vi "setUp.vi"(8 "error in (no error)":errorcluster, 11 "TestConfigurationFileBinding In":refnum<class "TestPersistToDiskTransport.lvclass">) -> (0 "error out":errorcluster, 3 "TestConfigurationFileBinding Out":refnum<class "TestPersistToDiskTransport.lvclass">)   [LabVIEW 2017, in "TestPersistToDiskTransport.lvclass"]
doc: "setUp runs prior to the test method during test execution. Use this method to initialize any object data required by your tests."
uses:
  TestPersistToDiskTransport.lvclass
  C:/Program Files (x86)/National Instruments/LabVIEW 2017/vi.lib/addons/_JKI Toolkits/VI Tester/TestCase.llb/TestCase.lvclass
  <vilib>/Utility/sysdir.llb/System Directory Type.ctl
  TestPersistToDiskTransport.lvclass/TestPersistToDiskTransport.ctl
  <vilib>/addons/_JKI Toolkits/VI Tester/TestCase.llb/TestCase.lvclass
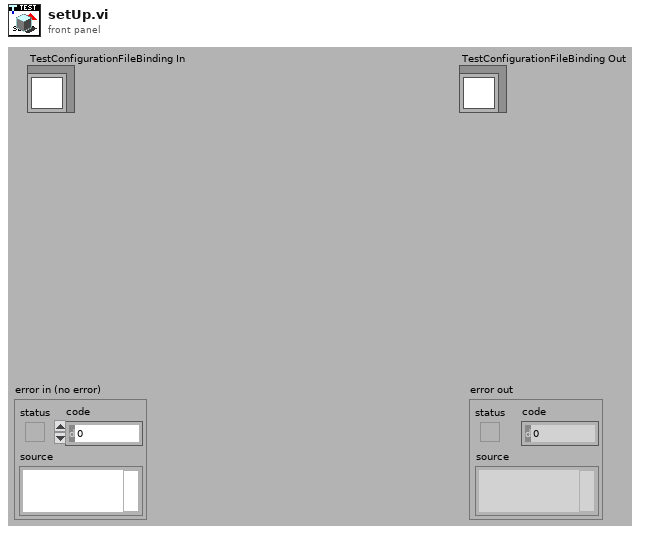
[diagram p1: front panel]
types:
  T1 = typedef "System Directory Type.ctl" = i32
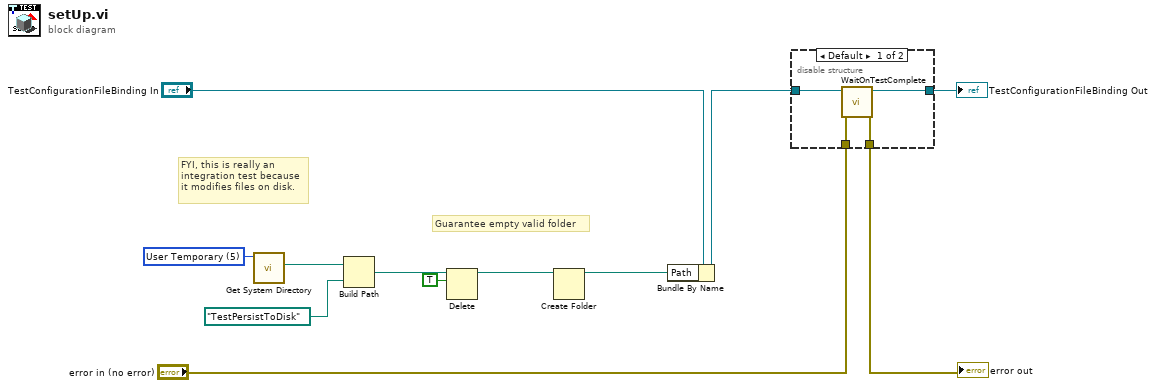
[diagram p0: block diagram]
diagram:
  w7 = T1 5 items=["User Home"=0, "User Desktop"=1, "User Documents"=2, "User Application Data"=3, "User Preferences"=4, "User Temporary"=5, "Public Documents"=6, "Public Application Data"=7, "Public Preferences"=8, "Public Cache"=13, "System Core Libraries"=9, "System Installed Libraries"=10, "Application Files"=11, "Boot Volume Root"=12] ("system directory type")
  # "Guarantee empty valid folder"
  # "FYI, this is really an\nintegration test because\nit modifies files on disk."
  n1 = call <vilib>:"Get System Directory.vi"("system directory type"=w7) -> ("system directory"=w6:path)  [unwired: 10 in]
  n2 = Build Path(base path=w6, name or relative path=path "TestPersistToDisk") -> (appended path=w4:path)
  n3 = Delete(path (use dialog)=w4, entire hierarchy (F)=TRUE) -> (deleted path=w2:path)  [unwired: 3 in, 2 out]
  n4 = Create Folder(path (use dialog)=w2) -> (created path=w3:path)  [unwired: 2 in, 2 out]
  n5 = Bundle By Name(cluster="TestConfigurationFileBinding In", "Path"=w3) -> (w8:refnum<class "TestPersistToDiskTransport.lvclass">)
  n6 = disable-structure shown="Default" {
    disable-tunnel: "error in (no error)" -> [w16 w17]
    disable-tunnel: [w15 w17] -> w11
    disable-tunnel: [w14 w18] -> w9
    disable-tunnel: w8 -> [w13 w18]
    frame condition #0 (active) {
      n7 = call <vilib>:"WaitOnTestComplete.vi"("error in (no error)"=w16, "TestCase in"=w13) -> ("error out"=w15:errorcluster, "TestCase out"=w14:refnum<class "TestPersistToDiskTransport.lvclass">)  [unwired: 8 in]
    }
    frame condition #1 {
    }
  }
  "error out" <- w11
  "TestConfigurationFileBinding Out" <- w9
